vi "Increment Score.vi"(8 "error in (no error)":errorcluster, 11 "Game Board in":refnum<class "Game Board.lvclass">) -> (0 "error out":errorcluster, 3 "Game Board out":refnum<class "Game Board.lvclass">)   [LabVIEW 2018, in "Game Board.lvclass"]
uses:
  Game Board.lvclass
  Game Board.lvclass/Game Board.ctl
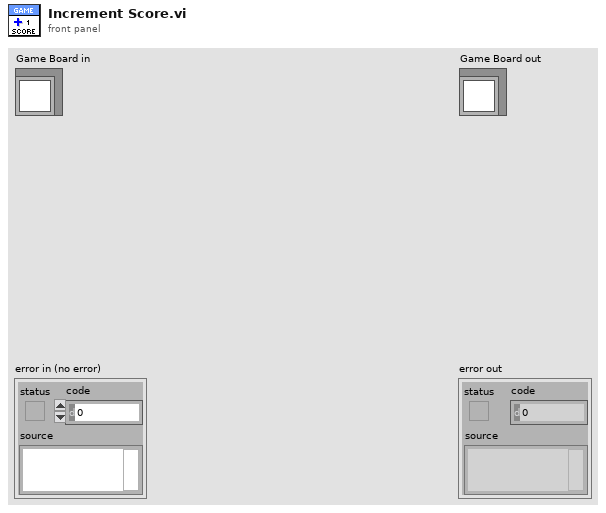
[diagram p1: front panel]
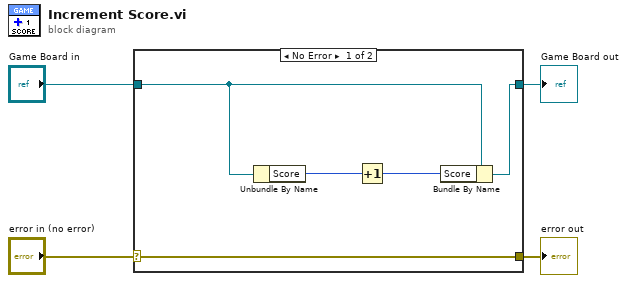
[diagram p0: block diagram]
diagram:
  n1 = case shown="No Error" "error in (no error)" {
    selector: "error in (no error)" -> [w9 w10]
    tunnel: [w9 w10] -> w3
    tunnel: [w8 w11] -> w1
    tunnel: "Game Board in" -> [w7 w11]
    frame No Error {
      n2 = Unbundle By Name(w7) -> ("Score"=w6:u32)
      n3 = Increment(x=w6) -> (x+1=w5:u32)
      n4 = Bundle By Name(cluster=w7, "Score"=w5) -> (w8:refnum<class "Game Board.lvclass">)
    }
    frame Error {
    }
  }
  "error out" <- w3
  "Game Board out" <- w1
